vi "__PW_read_and_preset.vi"(8 "MAXChiA,B,C,Dj":string="A", 11 "GPIB":string="3") -> ()   [LabVIEW 2017]
panel:
  out "ADmoni":dbl
  out "VDmoni":dbl
  out "ACmoni":dbl
  out "VCmoni":dbl
  out "ABmoni":dbl
  out "VBmoni":dbl
  out "AAmoni":dbl
  out "VAmoni":dbl
  out "•¶Žš—ñ":string="VA0.00,AA0.90"
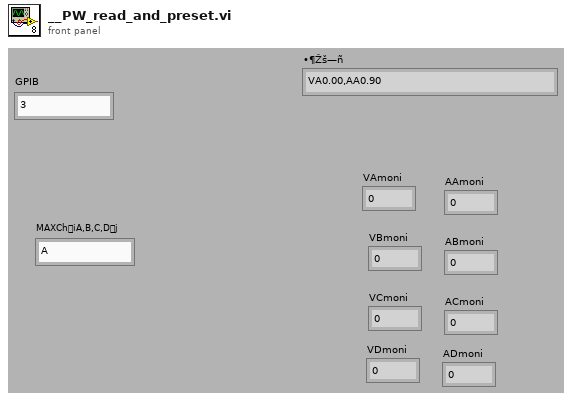
[diagram p1: front panel]
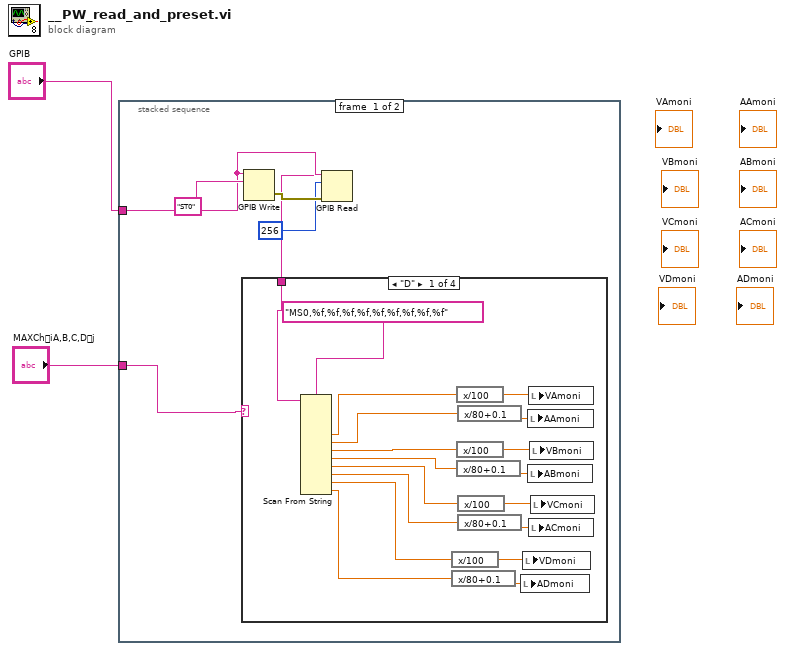
[diagram p0: block diagram]
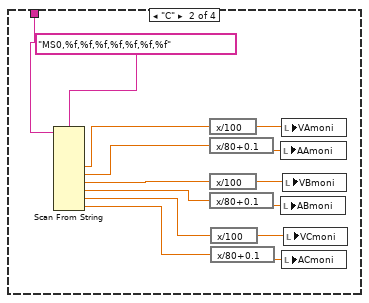
[diagram p2: hidden frame]
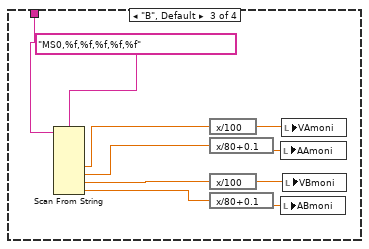
[diagram p3: hidden frame]
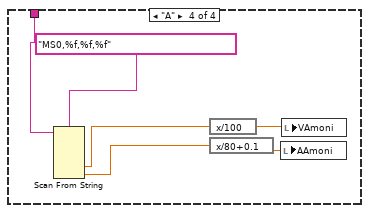
[diagram p4: hidden frame]
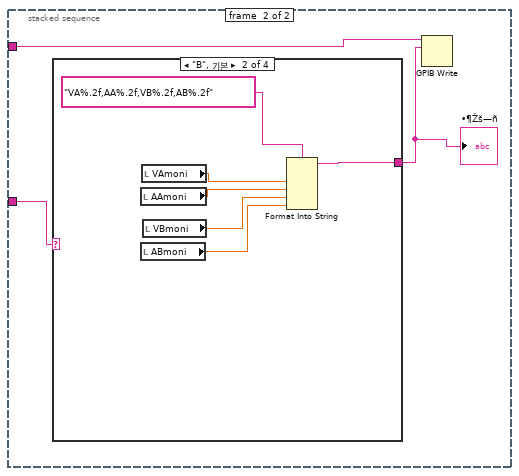
[diagram p5: hidden frame]
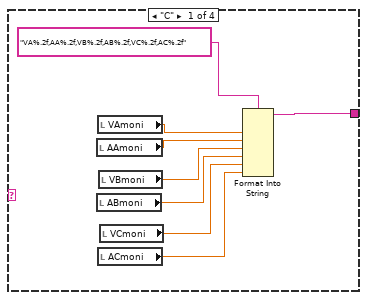
[diagram p6: hidden frame]
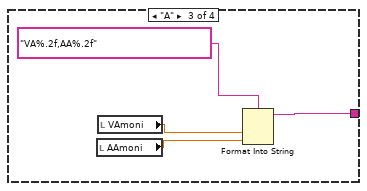
[diagram p7: hidden frame]
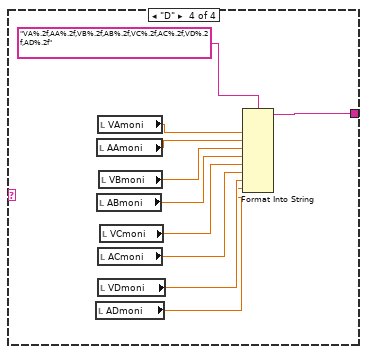
[diagram p8: hidden frame]
diagram:
  n1 = stacked-sequence {
    tunnel: "GPIB" -> [w6 w59]
    tunnel: "MAXChiA,B,C,Dj" -> [w3 w58]
    frame #0 {
      n2 = GPIB Write(0:w6, 1:"ST0") -> (6:w7:errorcluster)  [unwired: 3 in, 1 out]
      n3 = GPIB Read(0:w6, 1:256, 3:w7) -> (5:w4:string)  [unwired: 2 in, 2 out]
      n4 = case shown="\"D\"" w3 {
        tunnel: w4 -> [w26 w40 w50 w56]
        frame "D" {
          n5 = Scan From String(format string="MS0,%f,%f,%f,%f,%f,%f,%f,%f,%f", input string=w26) -> (output 2=w11:dbl, output 3=w10:dbl, output 4=w9:dbl, output 5=w12:dbl, output 6=w18:dbl, output 7=w17:dbl, output 8=w23:dbl, output 9=w24:dbl)  [unwired: 12 in, 3 out]
          n6 = expression code="x/100"(w23) -> (w22:dbl)
          n7 = expression code="x/80+0.1"(w24) -> (w21:dbl)
          n8 = expression code="x/100"(w11) -> (w13:dbl)
          n9 = expression code="x/100"(w9) -> (w16:dbl)
          n10 = expression code="x/80+0.1"(w12) -> (w15:dbl)
          n11 = expression code="x/80+0.1"(w10) -> (w14:dbl)
          n12 = expression code="x/100"(w18) -> (w19:dbl)
          n13 = expression code="x/80+0.1"(w17) -> (w20:dbl)
          n14 = local write "ADmoni"(w21) -> ()
          n15 = local write "VDmoni"(w22) -> ()
          n16 = local write "AAmoni"(w14) -> ()
          n17 = local write "ABmoni"(w15) -> ()
          n18 = local write "VAmoni"(w13) -> ()
          n19 = local write "ACmoni"(w20) -> ()
          n20 = local write "VBmoni"(w16) -> ()
          n21 = local write "VCmoni"(w19) -> ()
        }
        frame "C" {
          n22 = Scan From String(format string="MS0,%f,%f,%f,%f,%f,%f,%f", input string=w40) -> (output 2=w29:dbl, output 3=w28:dbl, output 4=w27:dbl, output 5=w30:dbl, output 6=w36:dbl, output 7=w35:dbl)  [unwired: 10 in, 3 out]
          n23 = expression code="x/100"(w29) -> (w31:dbl)
          n24 = expression code="x/80+0.1"(w28) -> (w32:dbl)
          n25 = expression code="x/100"(w27) -> (w34:dbl)
          n26 = expression code="x/80+0.1"(w30) -> (w33:dbl)
          n27 = expression code="x/100"(w36) -> (w37:dbl)
          n28 = expression code="x/80+0.1"(w35) -> (w38:dbl)
          n29 = local write "AAmoni"(w32) -> ()
          n30 = local write "ABmoni"(w33) -> ()
          n31 = local write "VAmoni"(w31) -> ()
          n32 = local write "ACmoni"(w38) -> ()
          n33 = local write "VBmoni"(w34) -> ()
          n34 = local write "VCmoni"(w37) -> ()
        }
        frame "B", Default {
          n35 = Scan From String(format string="MS0,%f,%f,%f,%f,%f", input string=w50) -> (output 2=w43:dbl, output 3=w42:dbl, output 4=w41:dbl, output 5=w44:dbl)  [unwired: 8 in, 3 out]
          n36 = expression code="x/100"(w43) -> (w45:dbl)
          n37 = expression code="x/80+0.1"(w42) -> (w46:dbl)
          n38 = expression code="x/100"(w41) -> (w48:dbl)
          n39 = expression code="x/80+0.1"(w44) -> (w47:dbl)
          n40 = local write "AAmoni"(w46) -> ()
          n41 = local write "ABmoni"(w47) -> ()
          n42 = local write "VAmoni"(w45) -> ()
          n43 = local write "VBmoni"(w48) -> ()
        }
        frame "A" {
          n44 = Scan From String(format string="MS0,%f,%f,%f", input string=w56) -> (output 2=w52:dbl, output 3=w51:dbl)  [unwired: 6 in, 3 out]
          n45 = expression code="x/100"(w52) -> (w53:dbl)
          n46 = expression code="x/80+0.1"(w51) -> (w54:dbl)
          n47 = local write "AAmoni"(w54) -> ()
          n48 = local write "VAmoni"(w53) -> ()
        }
      }
    }
    frame #1 {
      n49 = case shown="\"B\", 기본" w58 {
        tunnel: [w67 w73 w77 w87] -> w57
        frame "C" {
          n50 = local read "AAmoni"() -> (w64:dbl)
          n51 = local read "ABmoni"() -> (w62:dbl)
          n52 = local read "VAmoni"() -> (w65:dbl)
          n53 = local read "ACmoni"() -> (w60:dbl)
          n54 = local read "VBmoni"() -> (w63:dbl)
          n55 = local read "VCmoni"() -> (w61:dbl)
          n56 = Format Into String(format string="VA%.2f,AA%.2f,VB%.2f,AB%.2f,VC%.2f,AC%.2f", w65, w64, w63, w62, w61, w60) -> (resulting string=w67:string)  [unwired: 2 in, 1 out]
        }
        frame "B", Default {
          n57 = local read "AAmoni"() -> (w70:dbl)
          n58 = local read "ABmoni"() -> (w68:dbl)
          n59 = local read "VAmoni"() -> (w71:dbl)
          n60 = local read "VBmoni"() -> (w69:dbl)
          n61 = Format Into String(format string="VA%.2f,AA%.2f,VB%.2f,AB%.2f", w71, w70, w69, w68) -> (resulting string=w73:string)  [unwired: 2 in, 1 out]
        }
        frame "A" {
          n62 = local read "AAmoni"() -> (w74:dbl)
          n63 = local read "VAmoni"() -> (w75:dbl)
          n64 = Format Into String(format string="VA%.2f,AA%.2f", w75, w74) -> (resulting string=w77:string)  [unwired: 2 in, 1 out]
        }
        frame "D" {
          n65 = local read "ADmoni"() -> (w78:dbl)
          n66 = local read "AAmoni"() -> (w84:dbl)
          n67 = local read "ABmoni"() -> (w82:dbl)
          n68 = local read "VAmoni"() -> (w85:dbl)
          n69 = local read "ACmoni"() -> (w80:dbl)
          n70 = local read "VDmoni"() -> (w79:dbl)
          n71 = local read "VBmoni"() -> (w83:dbl)
          n72 = local read "VCmoni"() -> (w81:dbl)
          n73 = Format Into String(format string="VA%.2f,AA%.2f,VB%.2f,AB%.2f,VC%.2f,AC%.2f,VD%.2f,AD%.2f", w85, w84, w83, w82, w81, w80, w79, w78) -> (resulting string=w87:string)  [unwired: 2 in, 1 out]
        }
      }
      "•¶Žš—ñ" <- w57
      n74 = GPIB Write(0:w59, 1:w57) -> ()  [unwired: 3 in, 2 out]
    }
  }
